vi "Drive Twist.vi"(11 "Cluster":T1) -> (3 "Cluster 2":T1)   [LabVIEW 2018]
uses:
  TypeDefs/Teleop Data Cluster.ctl
  TypeDefs/Joystick Axes.ctl
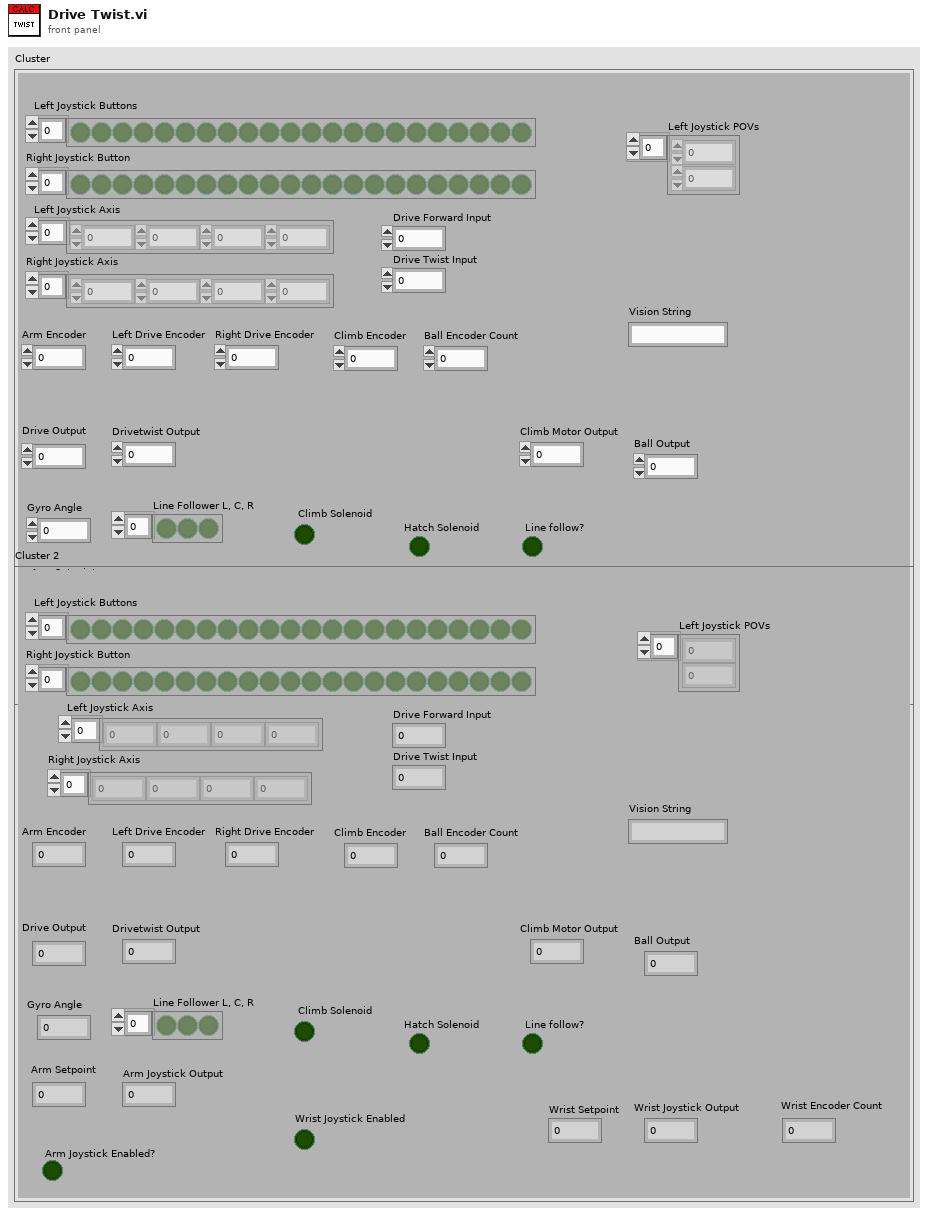
[diagram p1: front panel]
types:
  T1 = typedef "Teleop Data Cluster.ctl" = cluster{"Drive Forward Input ":dbl, "Drive Twist Input":dbl, "Drive Output":dbl, "Drivetwist Output":dbl, "Left Joystick Buttons":bool[], "Left Joystick Axis":dbl[], "Right Joystick Axis":dbl[], "Right Joystick Button":bool[], "Arm Encoder":dbl, "Left Drive Encoder":dbl, "Right Drive Encoder":dbl, "Gyro Angle ":dbl, "Arm Joystick Output  ":dbl, "Line Follower L, C, R ":bool[], "Line follow?":bool, " Climb Solenoid":bool, "Wrist Encoder Count":dbl, "Wrist Joystick Output":dbl, "Ball Encoder Count":dbl, "Ball Output":dbl, "Climb Encoder":dbl, "Climb Motor Output":dbl, " Hatch Solenoid":bool, "Arm Setpoint ":dbl, "Wrist Setpoint ":dbl, "Arm Joystick Enabled?":bool, "Wrist Joystick Enabled":bool, "Vision String":string, "Left Joystick POVs":i16[]}
  T2 = typedef "Joystick Axes.ctl" = enum16{"X Axis", "Y Axis", "Twist Axis", "Throttle"}
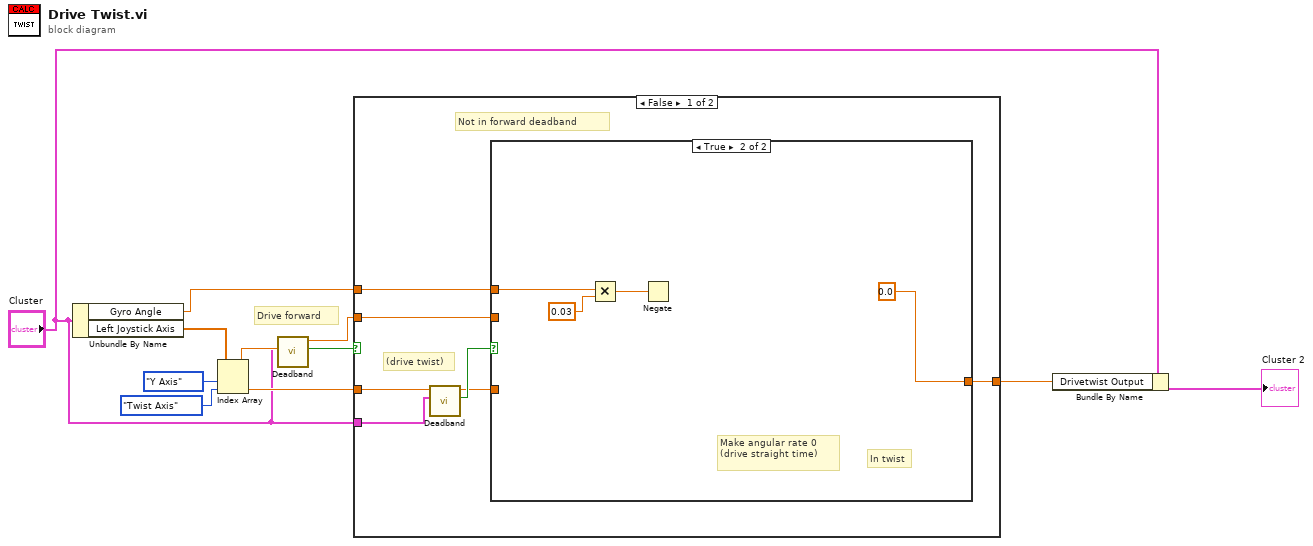
[diagram p0: block diagram]
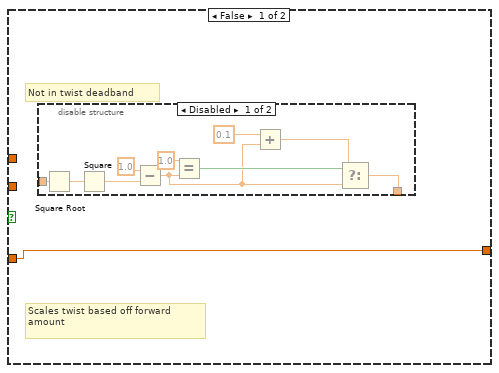
[diagram p2: hidden frame]
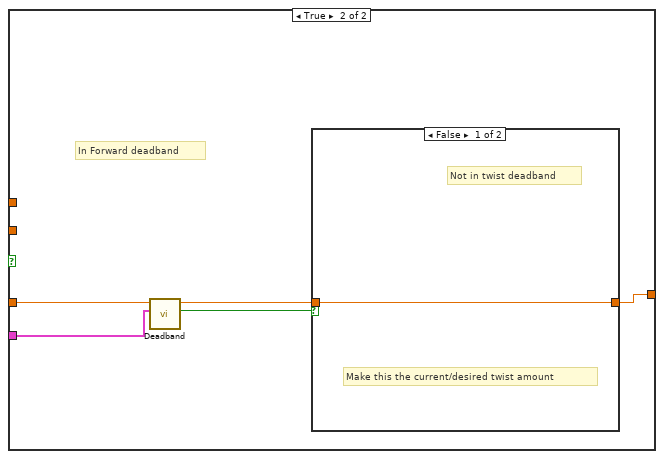
[diagram p4: hidden frame]
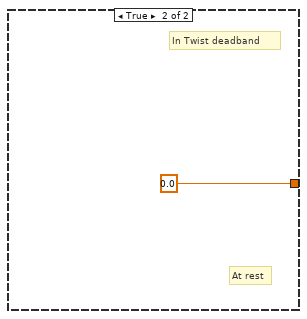
[diagram p5: hidden frame]
diagram:
  # "Drive forward"
  n1 = Unbundle By Name("Cluster") -> ("Gyro Angle"=w2:dbl, "Left Joystick Axis"=w11:dbl[])
  n2 = Index Array(array=w11, index #1=Joystick_Axes."Y Axis" ("Enum"), index #2=Joystick_Axes."Twist Axis" ("Enum")) -> (element #1=w8:dbl, element #2=w6:dbl)
  n3 = call "Deadband.vi"("Cluster"="Cluster", "Twiest Input"=w8) -> ("Dead Band Zone"=w7:bool, "Tweest Interpreted"=w3:dbl)  [unwired: 8 in]
  n4 = case shown="False" w7 {
    tunnel: w6 -> [w18 w38]
    tunnel: [w16 w36] -> w4
    tunnel: w3 -> [w14 _]
    tunnel: w2 -> [w13 _]
    tunnel: "Cluster" -> [w12 w34]
    frame False {
      # "(drive twist)"
      # "Not in forward deadband"
      n5 = call "Deadband.vi"("Cluster"=w12, "Twiest Input"=w18) -> ("Dead Band Zone"=w17:bool, "Tweest Interpreted"=w15:dbl)  [unwired: 8 in]
      n6 = case shown="True" w17 {
        tunnel: [w19 0.0 ("Foward Interpreted")] -> w16
        tunnel: w15 -> [w19 _]
        tunnel: w14 -> [_ _]
        tunnel: w13 -> [_ w33]
        frame False {
          # "Scales twist based off forward\namount"
          # "Not in twist deadband"
          n7 = disable-structure shown="Disabled" {
            disable-tunnel: [w28 _] -> _
            disable-tunnel: _ -> [w22 _]
            frame Disabled {
              n8 = Square Root(x=w22) -> (sqrt(x)=w21:dbl)
              n9 = Square(x=w21) -> (x^2=w20:dbl)
              n10 = Subtract(x=1.0, y=w20) -> (x-y=w25:dbl)
              n11 = Equal?(x=1.0, y=w25) -> (x = y?=w26:bool)
              n12 = Add(x=0.1, y=w25) -> (x+y=w23:dbl)
              n13 = Select(t=w23, s=w26, f=w25) -> (s? t:f=w28:dbl)
            }
            frame Enabled {
            }
          }
        }
        frame True {
          # "Make angular rate 0\n(drive straight time)"
          # "In twist"
          n14 = Multiply(x=w33, y=0.03) -> (x*y=w31:dbl)
          n15 = Negate(x=w31) -> ()  [unwired: 1 out]
        }
      }
    }
    frame True {
      # "In Forward deadband"
      n16 = call "Deadband.vi"("Cluster"=w34, "Twiest Input"=w38) -> ("Dead Band Zone"=w37:bool, "Tweest Interpreted"=w35:dbl)  [unwired: 8 in]
      n17 = case shown="False" w37 {
        tunnel: [w39 0.0] -> w36
        tunnel: w35 -> [w39 _]
        frame False {
          # "Make this the current/desired twist amount"
          # "Not in twist deadband"
        }
        frame True {
          # "At rest"
          # "In Twist deadband"
        }
      }
    }
  }
  n18 = Bundle By Name(cluster="Cluster", "Drivetwist Output"=w4) -> (→"Cluster 2":T1)
